vi "Serial Number (Read).vi"(6 "ISOBUS address":T2=-1 caption="ISOBUS address (-1)", 8 "error in":errorcluster, 11 "Mercury Reference In":T3) -> (0 "error out":errorcluster, 2 "Serial Number":string, 3 "Mercury Reference Out":T3, 4 "Valid?":T1)   [LabVIEW 2013, in "Mercury iXX.lvlib" / "Heater.lvlib"]
doc: "Returns the serial number of the selected heater device."
uses:
  Heater.lvlib
  Mercury iXX.lvlib
  Private/Controls/Command Verbs.ctl
  Controls/Comms Transport Layer.ctl
  Controls/Mercury Reference.ctl
  Controls/Is Valid LED.ctl
  Controls/ISOBus Address.ctl
  Private/Controls/Query Dynamic Reference.ctl
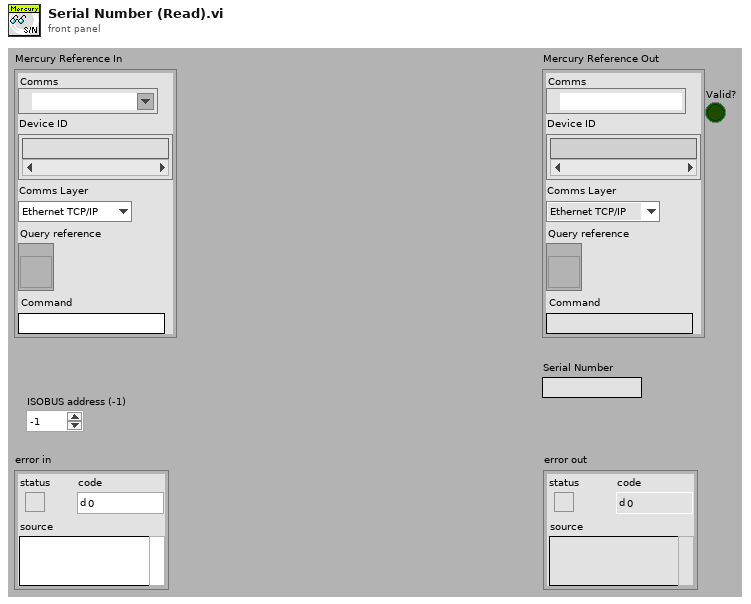
[diagram p1: front panel]
types:
  T1 = typedef "Mercury iXX.lvlib/Is Valid LED.ctl" = bool
  T2 = typedef "Mercury iXX.lvlib/ISOBus Address.ctl" = i32
  T3 = typedef "Mercury iXX.lvlib/Mercury Reference.ctl" = cluster{"Comms":refnum<visa-resource-name>, "Device ID":string[], "Comms Layer":T4, "Command":string, "Query reference":T5}
  T4 = typedef "Mercury iXX.lvlib/Comms Transport Layer.ctl" = enum16{"Ethernet TCP/IP", "USB", "ISOBus - RS-232", "GPIB"}
  T5 = typedef "Mercury iXX.lvlib/Query Dynamic Reference.ctl" = refnum<vi>
  T6 = typedef "Mercury iXX.lvlib/Command Verbs.ctl" = string
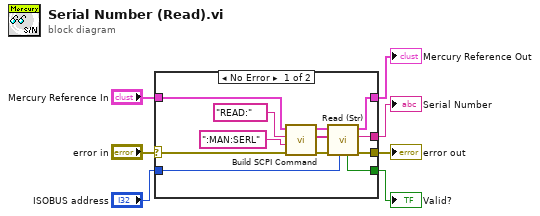
[diagram p0: block diagram]
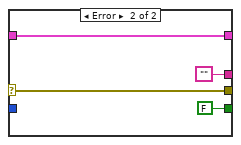
[diagram p2: hidden frame]
diagram:
  n1 = case shown="No Error" "error in" {
    selector: "error in" -> [w9 w22]
    tunnel: "Mercury Reference In" -> [w10 w23]
    tunnel: [w15 w23] -> w6
    tunnel: [w14 w22] -> w5
    tunnel: "ISOBUS address" -> [w11 _]
    tunnel: [w13 ""] -> w2
    tunnel: [w12 FALSE ("Valid?")] -> w1
    frame No Error {
      n2 = call "Build SCPI Command.vi"("error in"=w9, "Noun(s)"=":MAN:SERL" ("Command"), "Verb"=T6 "READ:", "Mercury Reference In"=w10) -> ("error out"=w19:errorcluster, "SCPI Message(s)"=w16:string[], "Mercury Reference Out"=w17:T3)  [unwired: 5 out]
      n3 = call "Read (Str).vi"("ISOBUS address"=w11, "error in"=w19, "SCPI Message(s)"=w16, "Mercury Reference In"=w17) -> ("error out"=w14:errorcluster, "Response"=w13:string, "Mercury Reference Out"=w15:T3, "Valid?"=w12:T1)  [unwired: 4 out]
    }
    frame Error {
    }
  }
  "Mercury Reference Out" <- w6
  "error out" <- w5
  "Serial Number" <- w2
  "Valid?" <- w1
